vi "LuaVIEW Open Base State.vi"(0 "close identifier (none)":string, 11 "error in (no error)":errorcluster) -> (6 "LuaVIEW reference":T1, 15 "error out":errorcluster)   [LabVIEW 2013]
doc: "Opens a LuaVIEW base state which is essentially an instance of the Lua virtual machine with associated storage, and returns a reference to it. A base state lacks the infrastructure and preparations required for calling LabVIEW from Lua. Instead it is intended for hosting functions to be called from LabVIEW via the \"Call\". To define callable functions, compile and execute a script containing function definitions for a base state.\n\nClosing a base state is not required when it is only opened once during an application run: open base states are closed when the LuaVIEW VIs unload. When repeatedly opening a state for the same purpose, the \"close identifier\" can be used to automatically close stale states."
uses:
  typedefs/t_LuaVIEW Reference.ctl
  typedefs/t_LuaVIEW CIN Spinlocked Actions.ctl
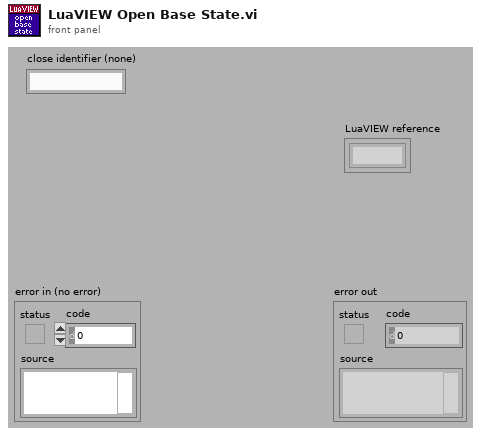
[diagram p1: front panel]
types:
  T1 = typedef "t_LuaVIEW Reference.ctl" = refnum<k1>
  T2 = typedef "t_LuaVIEW CIN Spinlocked Actions.ctl" = enum16{"totals", "taskcount", "open", "registerpublic", "registerexport", "revokeexports", "unregnextpublic", "usepublic", "pollexport", "close", "startyieldtest", "endyieldtest", "pollprintbuffer"}
  T3 = typedef "et_LuaVIEW CIN Results.ctl" = enum16{"OK", "error", "main", "call", "clonecall", "modulecall", "exportcall", "index", "yield"}
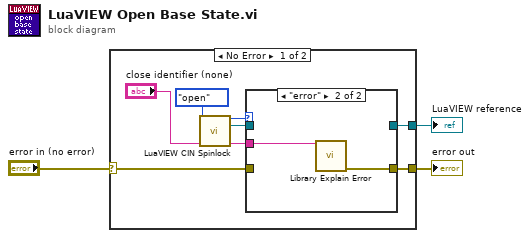
[diagram p0: block diagram]
diagram:
  n1 = case shown="No Error" "error in (no error)" {
    selector: "error in (no error)" -> [w7 w16]
    tunnel: [w8 w16] -> w1
    tunnel: [w6 _] -> w2
    frame No Error {
      n2 = call "LuaVIEW CIN Spinlock.vi"("action"=t_LuaVIEW_CIN_Spinlocked_Actions."open", "string in"="close identifier (none)") -> ("result"=w11:T3, "LuaVIEW reference out"=w9:T1, "string out"=w10:string)  [unwired: 7 in, 4 out]
      n3 = case shown="\"error\"" w11 {
        tunnel: w10 -> [_ w15]
        tunnel: w9 -> [w13 _]
        tunnel: [w13 _] -> w6
        tunnel: [w12 w14] -> w8
        tunnel: w7 -> [w12 _]
        frame Default {
        }
        frame "error" {
          n4 = call "Library Explain Error.vi"("explanation prefix (none)"=w15) -> ("explained error"=w14:errorcluster)  [unwired: 14 in]
        }
      }
    }
    frame Error {
    }
  }
  "LuaVIEW reference" <- w2
  "error out" <- w1
